vi "Software Update HCC Header Search.vi"(10 "Input Data":string[][](array[string]), 11 "Station And Board ID Paths":path) -> (3 "Updated Input":string[][](array[string]))   [LabVIEW 2016]
uses:
  <vilib>/Utility/file.llb/Write To Spreadsheet File (string).vi
panel:
  out "Found Current Header":bool
  out "Found Agilent Header":bool
  out "Original Input":string[](array[string])
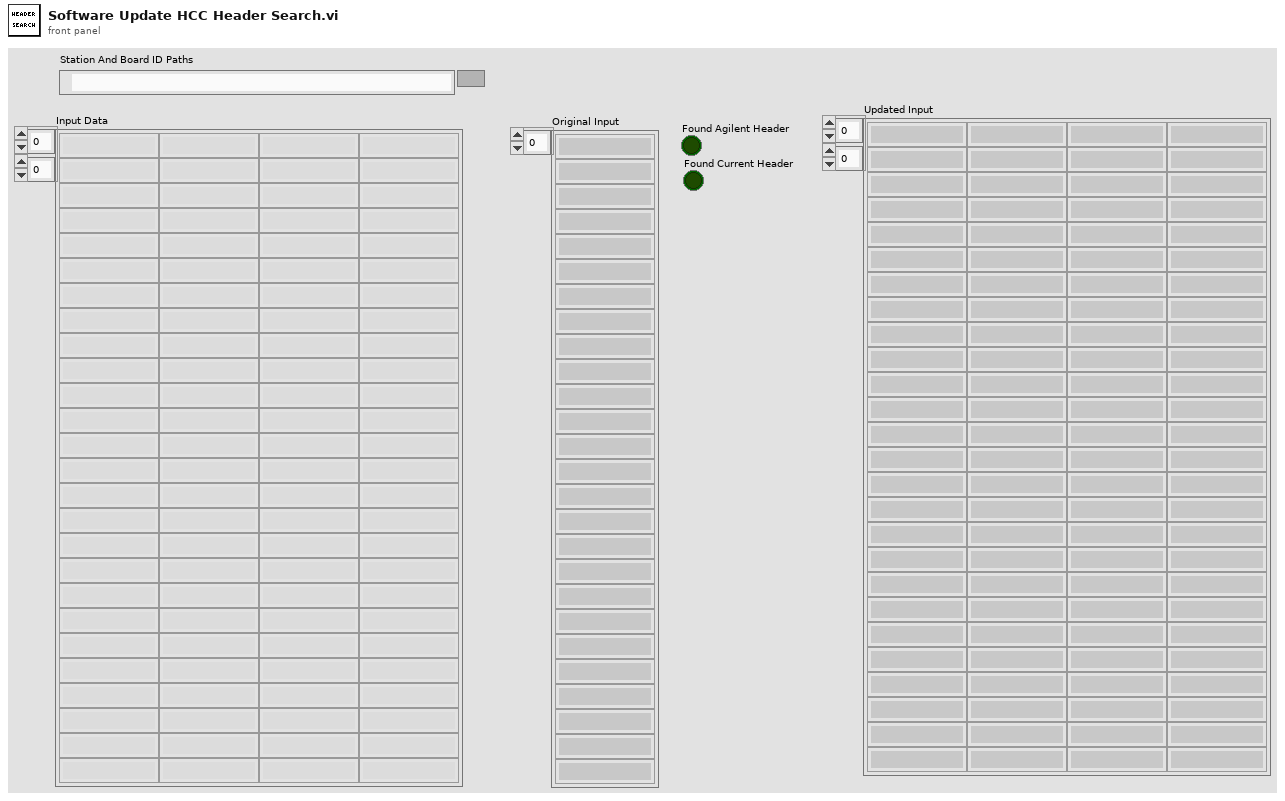
[diagram p1: front panel]
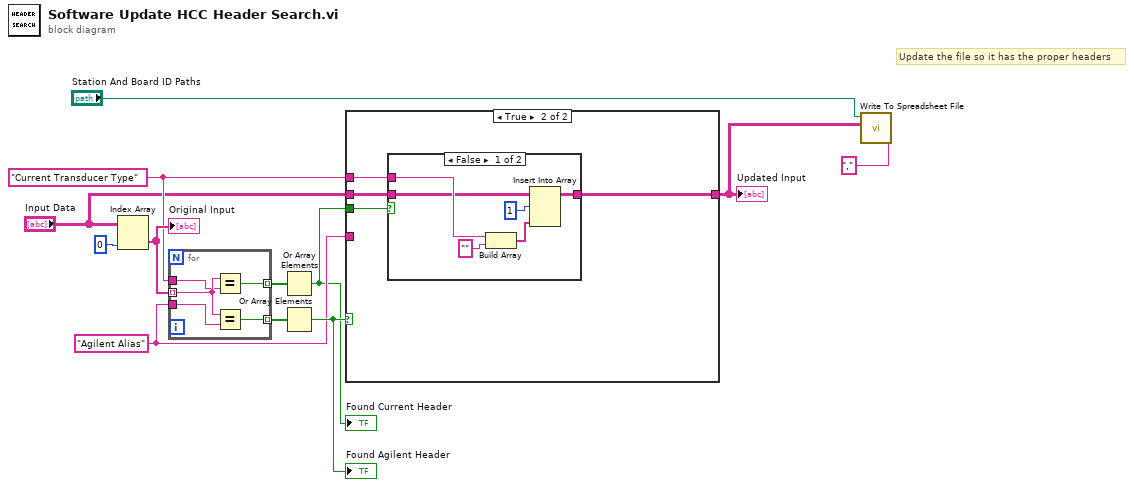
[diagram p0: block diagram]
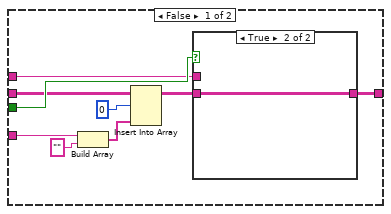
[diagram p2: hidden frame]
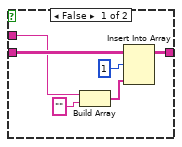
[diagram p3: hidden frame]
diagram:
  w6 = "Current Transducer Type"
  w7 = "Agilent Alias"
  # "Update the file so it has the proper headers"
  n1 = Index Array(array="Input Data", index (col)=0 ("disabled index (col)")) -> (element=w8:string[])  [unwired: 1 in]
  "Original Input" <- w8
  n2 = for {
    tunnel: w8 -> [w17] mode=indexing
    tunnel: [w16] -> w10 mode=indexing
    tunnel: [w15] -> w11 mode=indexing
    tunnel: w7 -> [w14]
    tunnel: w6 -> [w13]
    n3 = Equal?(x=w17, y=w13) -> (x = y?=w15:bool)
    n4 = Equal?(x=w17, y=w14) -> (x = y?=w16:bool)
  }
  n5 = Or Array Elements(Boolean array=w11) -> (logical OR=w5:bool)
  "Found Current Header" <- w5
  n6 = Or Array Elements(Boolean array=w10) -> (logical OR=w9:bool)
  "Found Agilent Header" <- w9
  n7 = case shown="True" w9 {
    tunnel: "Input Data" -> [w21 w37]
    tunnel: w7 -> [w26 _]
    tunnel: w6 -> [w20 w35]
    tunnel: w5 -> [w22 w36]
    tunnel: [w18 w34] -> w2
    frame False {
      n8 = Build Array(w26, "") -> (w24:string[])
      n9 = Insert Into Array(array=w21, index (row)=0 ("index"), new element=w24) -> (w19:string[][])  [unwired: 1 in]
      n10 = case shown="True" w22 {
        tunnel: w19 -> [w29 w33]
        tunnel: w20 -> [w28 _]
        tunnel: [w27 w33] -> w18
        frame False {
          n11 = Build Array(w28, "") -> (w31:string[])
          n12 = Insert Into Array(array=w29, index (row)=1 ("index"), new element=w31) -> (w27:string[][])  [unwired: 1 in]
        }
        frame True {
        }
      }
    }
    frame True {
      n13 = case shown="False" w36 {
        tunnel: w37 -> [w39 w44]
        tunnel: w35 -> [w41 _]
        tunnel: [w40 w44] -> w34
        frame False {
          n14 = Build Array(w41, "") -> (w38:string[])
          n15 = Insert Into Array(array=w39, index (row)=1 ("index"), new element=w38) -> (w40:string[][])  [unwired: 1 in]
        }
        frame True {
        }
      }
    }
  }
  "Updated Input" <- w2
  n16 = call-poly <vilib>:"Write To Spreadsheet File.vi"("delimiter (\\t)"="," ("delimiter (\\t)"), "2D data"=w2, "file path (dialog if empty)"="Station And Board ID Paths") -> ()  [unwired: 5 in, 1 out]
